vi "PC_Main2.vi"() -> ()   [LabVIEW 2017]
uses:
  <vilib>/userdefined/High Color/IMAQdx.ctl
  pc_state.ctl
  <vilib>/vision/NI_Vision_Development_Module.lvlib
panel:
  out "Session Out":T1(plugin-control)
  in  "Camera Source":T2="cam1"
  in  "stop":bool
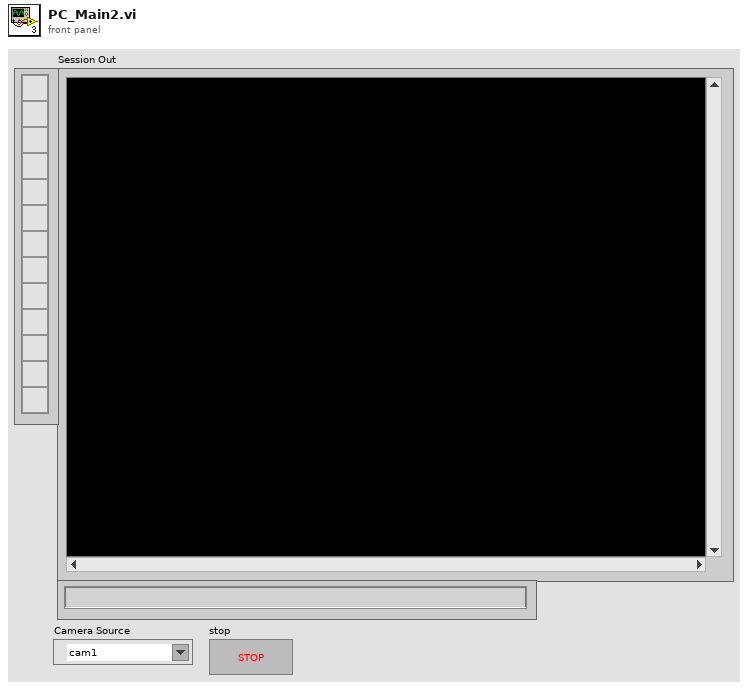
[diagram p1: front panel]
types:
  T1 = typedef "IMAQ Image.ctl" = refnum<image>
  T2 = typedef "IMAQdx.ctl" = refnum<k21>
  T3 = typedef "pc_state.ctl" = enum16{"Aquire Still Image", "Calibrate Image", "Increment State", "Stop", "Save Grid Image", "Save Table Image", "Threshold Image", "Remove Border"}
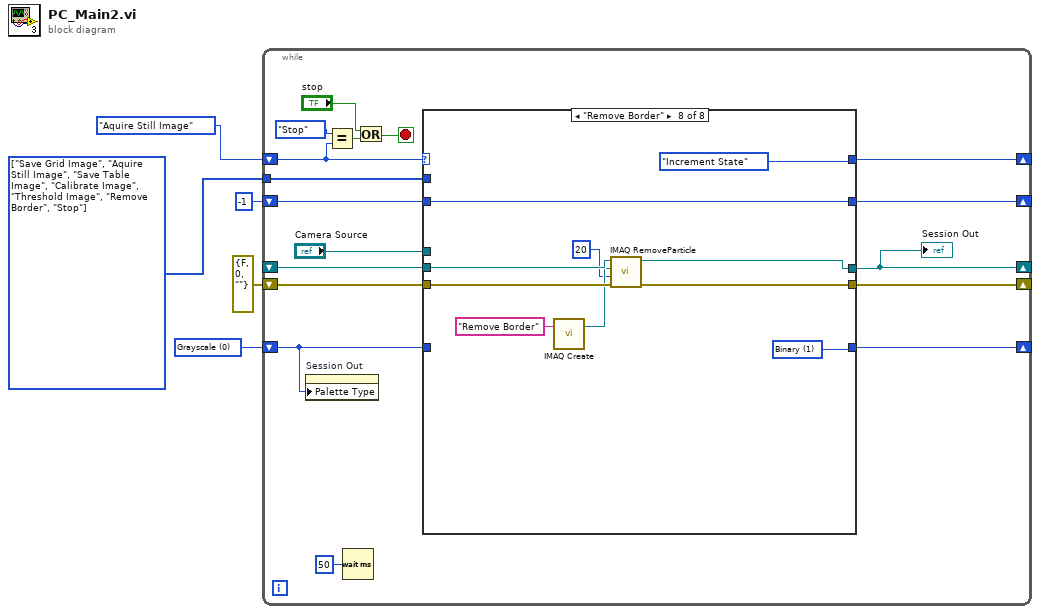
[diagram p0: block diagram]
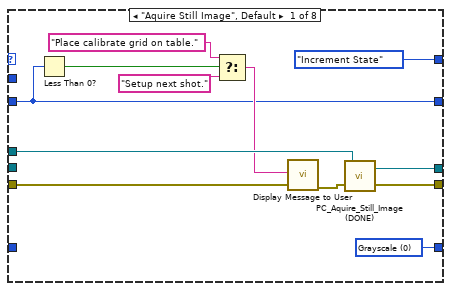
[diagram p2: hidden frame]
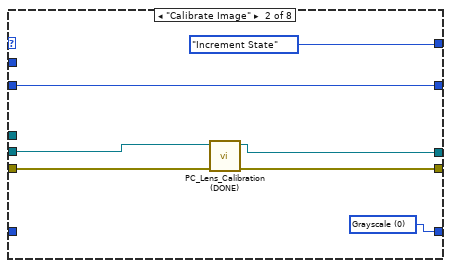
[diagram p3: hidden frame]
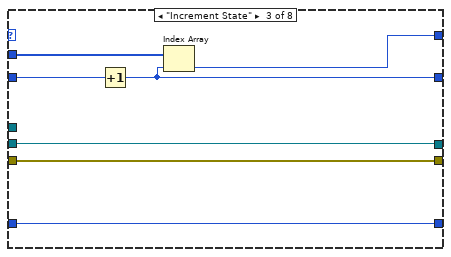
[diagram p4: hidden frame]
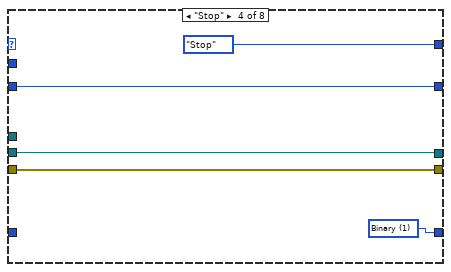
[diagram p5: hidden frame]
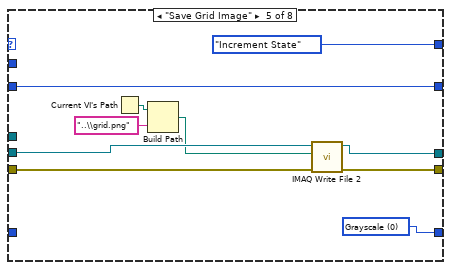
[diagram p6: hidden frame]
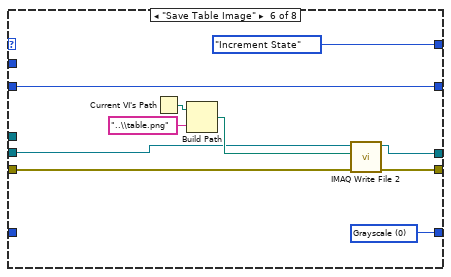
[diagram p7: hidden frame]
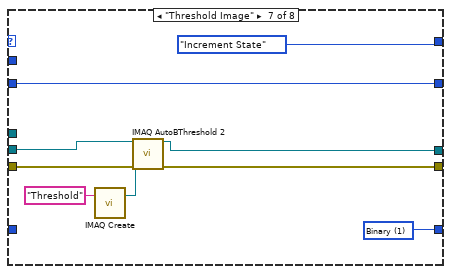
[diagram p8: hidden frame]
diagram:
  w1 = u32 0 items=["Grayscale", "Binary", "Gradient", "Rainbow", "Temperature", "User Defined", "Binary 16 Bit", "Gradient 16 Bit", "Rainbow 16 Bit", "Temperature 16 Bit", "User Defined 16 Bit"] ("Palette:Palette Type")
  w4 = T3[] [enum."Save Grid Image", enum."Aquire Still Image", enum."Save Table Image", enum."Calibrate Image", enum."Threshold Image", enum."Remove Border", enum."Stop"] items=["Aquire Still Image", "Calibrate Image", "Increment State", "Stop", "Save Grid Image", "Save Table Image", "Threshold Image", "Remove Border"]
  n1 = while {
    shift-right: [w22] -> _
    shift-left: errorcluster {"status"=FALSE, "code"=0, "source"=""} ("error out") -> [w21]
    shift-right: [w19] -> _
    shift-left: _ -> [w18]
    shift-right: [w14] -> _
    shift-left: pc_state."Aquire Still Image" -> [w9]
    tunnel: w4 -> [w16]
    shift-right: [w13] -> _
    shift-left: -1 -> [w15]
    shift-right: [w7] -> _
    shift-left: w1 -> [w6]
    stop <- w10 stop-if-true
    n2 = property on="Session Out" class="ImageControl"("Palette Type"=w6) -> ()  [unwired: 2 in, 2 out]
    n3 = Equal?(x=pc_state."Stop", y=w9) -> (x = y?=w12:bool)
    n4 = Wait (ms)(milliseconds to wait=u32 50) -> ()  [unwired: 1 out]
    n5 = Or(x="stop", y=w12) -> (x .or. y?=w10:bool)
    n6 = case shown="\"Remove Border\"" w9 {
      tunnel: [w34 w36 w44 w53 w60 w66 w78 w83] -> w19
      tunnel: [w33 w38 w43 w52 w61 w67 w80 w87] -> w22
      tunnel: w21 -> [w24 w39 w43 w52 w62 w69 w81 w88]
      tunnel: "Camera Source" -> [w32 _ _ _ _ _ _ _]
      tunnel: w18 -> [_ w37 w44 w53 w59 w68 w79 w86]
      tunnel: w16 -> [_ _ w47 _ _ _ _ _]
      tunnel: w15 -> [w28 w41 w48 w51 w63 w73 w82 w92]
      tunnel: [pc_state."Increment State" pc_state."Increment State" w46 pc_state."Stop" pc_state."Increment State" pc_state."Increment State" pc_state."Increment State" pc_state."Increment State"] -> w14
      tunnel: [w28 w41 w45 w51 w63 w73 w82 w92] -> w13
      tunnel: [w23 w35 w42 w49 w54 w64 w74 w89] -> w7
      tunnel: w6 -> [_ _ w42 _ _ _ _ _]
      frame "Aquire Still Image", Default {
        w23 = u32 0 items=["Grayscale", "Binary", "Gradient", "Rainbow", "Temperature", "User Defined", "Binary 16 Bit", "Gradient 16 Bit", "Rainbow 16 Bit", "Temperature 16 Bit", "User Defined 16 Bit"] ("Palette:Palette Type")
        n7 = Less Than 0?(x=w28) -> (x < 0?=w29:bool)
        n8 = Select(t="Place calibrate grid on table.", s=w29, f="Setup next shot.") -> (s? t:f=w30:string)
        n9 = call "Display Message to User"("error in (no error)"=w24, "Message"=w30) -> ("error out"=w25:errorcluster)  [unwired: 8 in, 1 out]
        n10 = call "PC_Aquire_Still_Image (DONE).vi"("Error In"=w25, "Camera Source"=w32) -> ("Error Out"=w33:errorcluster, "Session Out"=w34:T1)
      }
      frame "Calibrate Image" {
        w35 = u32 0 items=["Grayscale", "Binary", "Gradient", "Rainbow", "Temperature", "User Defined", "Binary 16 Bit", "Gradient 16 Bit", "Rainbow 16 Bit", "Temperature 16 Bit", "User Defined 16 Bit"] ("Palette:Palette Type")
        n11 = call "PC_Lens_Calibration (DONE).vi"("Error In"=w39, "Image In"=w37) -> ("Error Out"=w38:errorcluster, "Calibrated Image"=w36:T1)  [unwired: 8 in]
      }
      frame "Increment State" {
        n12 = Increment(x=w48) -> (x+1=w45:i32)
        n13 = Index Array(array=w47, index=w45) -> (element=w46:T3)
      }
      frame "Stop" {
        w49 = u32 1 items=["Grayscale", "Binary", "Gradient", "Rainbow", "Temperature", "User Defined", "Binary 16 Bit", "Gradient 16 Bit", "Rainbow 16 Bit", "Temperature 16 Bit", "User Defined 16 Bit"] ("Palette:Palette Type")
      }
      frame "Save Grid Image" {
        w54 = u32 0 items=["Grayscale", "Binary", "Gradient", "Rainbow", "Temperature", "User Defined", "Binary 16 Bit", "Gradient 16 Bit", "Rainbow 16 Bit", "Temperature 16 Bit", "User Defined 16 Bit"] ("Palette:Palette Type")
        n14 = Current VI's Path() -> (path=w57:path)
        n15 = Build Path(base path=w57, name or relative path="..\\grid.png") -> (appended path=w55:path)
        n16 = call-poly "IMAQ Write File 2"("error in (no error)"=w62, "File Path"=w55, "Image"=w59) -> ("error out"=w61:errorcluster, "Image Out (duplicate)"=w60:T1)  [unwired: 7 in]
      }
      frame "Save Table Image" {
        w64 = u32 0 items=["Grayscale", "Binary", "Gradient", "Rainbow", "Temperature", "User Defined", "Binary 16 Bit", "Gradient 16 Bit", "Rainbow 16 Bit", "Temperature 16 Bit", "User Defined 16 Bit"] ("Palette:Palette Type")
        n17 = Current VI's Path() -> (path=w65:path)
        n18 = Build Path(base path=w65, name or relative path="..\\table.png") -> (appended path=w71:path)
        n19 = call-poly "IMAQ Write File 2"("error in (no error)"=w69, "File Path"=w71, "Image"=w68) -> ("error out"=w67:errorcluster, "Image Out (duplicate)"=w66:T1)  [unwired: 7 in]
      }
      frame "Threshold Image" {
        w74 = u32 1 items=["Grayscale", "Binary", "Gradient", "Rainbow", "Temperature", "User Defined", "Binary 16 Bit", "Gradient 16 Bit", "Rainbow 16 Bit", "Temperature 16 Bit", "User Defined 16 Bit"] ("Palette:Palette Type")
        n20 = call "IMAQ Create"("Image Name"="Threshold") -> ("New Image"=w76:T1)  [unwired: 4 in, 1 out]
        n21 = call "IMAQ AutoBThreshold 2"("Image Src"=w79, "Image Dst"=w76, "error in (no error)"=w81) -> ("Image Dst Out"=w78:T1, "error out"=w80:errorcluster)  [unwired: 10 in, 1 out]
      }
      frame "Remove Border" {
        w89 = u32 1 items=["Grayscale", "Binary", "Gradient", "Rainbow", "Temperature", "User Defined", "Binary 16 Bit", "Gradient 16 Bit", "Rainbow 16 Bit", "Temperature 16 Bit", "User Defined 16 Bit"] ("Palette:Palette Type")
        n22 = call "IMAQ Create"("Image Name"="Remove Border") -> ("New Image"=w85:T1)  [unwired: 4 in, 1 out]
        n23 = call "IMAQ RemoveParticle"("error in (no error)"=w88, "Number of Erosion"=20, "Image Dst"=w85, "Image Src"=w86) -> ("error out"=w87:errorcluster, "Image Dst Out"=w83:T1)  [unwired: 6 in]
      }
    }
    "Session Out" <- w19
  }
